vi "Control Digital IO Pin.vi"(8 "error in (no error)":errorcluster, 9 "Pin Value":bool, 10 "Pin Index":u8 format="%x", 11 "Refnum In":refnum<vi>) -> (0 "error out":errorcluster, 1 "Pin Value Out":bool, 2 "Pin Index Out":u8, 3 "Refnum Out":refnum<vi>)   [LabVIEW 2020, in "FirmataClient.lvlib"]
doc: "Allows requesting the state of a digital pin."
uses:
  FirmataClient.lvlib
  Controls/FirmataPinModes.ctl
panel:
  out "Pin Mode":T1=enum."Extended.DHT"
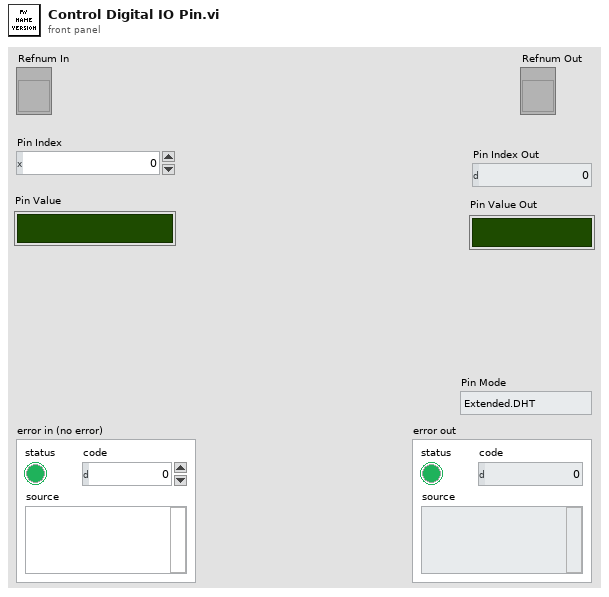
[diagram p1: front panel]
types:
  T1 = typedef "FirmataClient.lvlib/FirmataPinModes.ctl" = enum16{"DigitalInput", "DigitalOutput", "AnalogInput", "PWM", "Servo", "Shift", "I2C", "OneWire", "Stepper", "Encoder", "Serial", "InputPullup", "Extended.SPI", "Extended.Sonar", "Extended.Tone", "Extended.DHT"}
  T2 = typedef "FirmataClient.lvlib/FirmataProtocolConstants.ctl" = u16
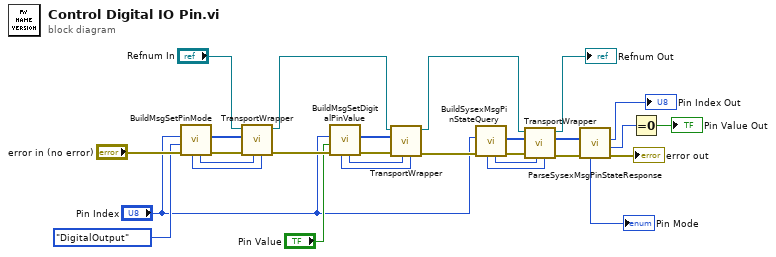
[diagram p0: block diagram]
diagram:
  n1 = call "BuildMsgSetPinMode.vi"("error in"="error in (no error)", "Pin Mode"=FirmataPinModes."DigitalOutput", "Pin Index"="Pin Index") -> ("error out"=w29:errorcluster, "SetPinModeMessage"=w24:u8[], "ReplyFirstByte"=w25:T2, "ReplyLength"=w26:i32)  [unwired: 5 in]
  n2 = call "TransportWrapper.vi"("ReplyLength"=w26, "ReplyFirstByte"=w25, "error in"=w29, "Message In"=w24, "Refnum In"="Refnum In") -> ("error out"=w18:errorcluster, "Refnum Out"=w17:refnum<vi>)  [unwired: 4 in, 1 out]
  n3 = call "BuildMsgSetDigitalPinValue.vi"("error in"=w18, "Pin Value"="Pin Value", "Pin Index"="Pin Index") -> ("error out"=w19:errorcluster, "DigitalPinValueMessage"=w22:u8[], "ReplyFirstByte"=w21:T2, "ReplyLength"=w20:i32)  [unwired: 5 in]
  n4 = call "TransportWrapper.vi"("ReplyLength"=w20, "ReplyFirstByte"=w21, "error in"=w19, "Message In"=w22, "Refnum In"=w17) -> ("error out"=w9:errorcluster, "Refnum Out"=w7:refnum<vi>)  [unwired: 4 in, 1 out]
  n5 = call "BuildSysexMsgPinStateQuery.vi"("error in"=w9, "Pin Index"="Pin Index") -> ("error out"=w15:errorcluster, "GetPinStateMessage"=w13:u8[], "ReplyFirstByte"=w11:T2, "ReplyLength"=w10:i32)  [unwired: 6 in]
  n6 = call "TransportWrapper.vi"("ReplyLength"=w10, "ReplyFirstByte"=w11, "error in"=w15, "Message In"=w13, "Refnum In"=w7) -> ("error out"=w14:errorcluster, "Message Out"=w12:u8[], "Refnum Out"=→"Refnum Out":refnum<vi>)  [unwired: 4 in]
  n7 = call "ParseSysexMsgPinStateResponse.vi"("error in"=w14, "Sysex Message"=w12) -> ("error out"=→"error out":errorcluster, "Pin State"=w2:u64, "Pin Index"=→"Pin Index Out":u8, "Pin Mode"=→"Pin Mode":T1)  [unwired: 6 in]
  n8 = Equal To 0?(x=w2) -> (x = 0?=→"Pin Value Out":bool)
